vi "5_VisualAD_HyperParam_Search.vi"() -> ()   [LabVIEW 2020]
uses:
  <vilib>/Ngene/DeepLTK Anomaly Detection Addon/DeepLTK_Anomaly_Detection_Addon/API/Controls/NNPC_Coreset_Params.ctl
  <vilib>/Ngene/DeepLTK Anomaly Detection Addon/DeepLTK_Anomaly_Detection_Addon/API/Controls/NNPC_Setup.ctl
  <vilib>/Ngene/Deep Learning Toolkit/Toolkit/NN_Data/API/NN_Dims(C,H,W).ctl
  <vilib>/Ngene/Deep Learning Toolkit/Toolkit/NN_Network/Controls/NN_Device.ctl
  <vilib>/Ngene/DeepLTK Anomaly Detection Addon/DeepLTK_Anomaly_Detection_Addon/API/Controls/Feature_Scorer_Params.ctl
  <vilib>/Ngene/DeepLTK Anomaly Detection Addon/DeepLTK_Anomaly_Detection_Addon/API/Controls/Gaussian_Blur.ctl
  <vilib>/Ngene/DeepLTK Anomaly Detection Addon/DeepLTK_Anomaly_Detection_Addon/API/Controls/Evaluation_Metrics.ctl
  <vilib>/Ngene/DeepLTK Anomaly Detection Addon/DeepLTK_Anomaly_Detection_Addon/API/Controls/Eval_Results.ctl
  <vilib>/Ngene/DeepLTK Anomaly Detection Addon/DeepLTK_Anomaly_Detection_Addon/API/Controls/MinMax.ctl
  <vilib>/Ngene/DeepLTK Anomaly Detection Addon/DeepLTK_Anomaly_Detection_Addon/API/Controls/NNPC_Random_Projection_CFG.ctl
  <vilib>/Ngene/DeepLTK Anomaly Detection Addon/DeepLTK_Anomaly_Detection_Addon/API/Controls/Dim_Reduction_Method.ctl
  <vilib>/Ngene/DeepLTK Anomaly Detection Addon/DeepLTK_Anomaly_Detection_Addon/API/Controls/NNFE_CFG.ctl
  <vilib>/Ngene/DeepLTK Anomaly Detection Addon/DeepLTK_Anomaly_Detection_Addon/API/Controls/Layer_Selector.ctl
  <vilib>/Ngene/DeepLTK Anomaly Detection Addon/DeepLTK_Anomaly_Detection_Addon/API/Controls/Feature_Layer_Selector.ctl
  <vilib>/Ngene/DeepLTK Anomaly Detection Addon/DeepLTK_Anomaly_Detection_Addon/API/Controls/Interpolation_Selector.ctl
  subVIs/Dataset_Reader/Controls/Read_Options.ctl
  <vilib>/Ngene/DeepLTK Anomaly Detection Addon/DeepLTK_Anomaly_Detection_Addon/API/Controls/NNPC_PreProcessing_Options.ctl
  <vilib>/Ngene/DeepLTK Anomaly Detection Addon/DeepLTK_Anomaly_Detection_Addon/API/Controls/NNPC_DS_Stats.ctl
  <vilib>/Ngene/DeepLTK Anomaly Detection Addon/DeepLTK_Anomaly_Detection_Addon/API/Controls/Image_Stats_RGB.ctl
  subVIs/HyperParam_Investigation/Controls/Model_Info_and_Report.ctl
  subVIs/HyperParam_Investigation/Controls/Feature_Layers_CFG.ctl
  <vilib>/Ngene/DeepLTK Anomaly Detection Addon/DeepLTK_Anomaly_Detection_Addon/API/Controls/Eval_Config.ctl
  <vilib>/Ngene/Deep Learning Toolkit/Toolkit/NN_Data/subVIs/Dataset_Destroy/NN_Dataset_Destroy(In3D_Out3D).vi
  <vilib>/Ngene/DeepLTK Anomaly Detection Addon/DeepLTK_Anomaly_Detection_Addon/API/Controls/NNPC_Save_CFG.ctl
  <vilib>/Ngene/DeepLTK Anomaly Detection Addon/DeepLTK_Anomaly_Detection_Addon/API/NNPC_Generate_Embedding/NNPC_Generate_Embedding(Dataset).vi
  <vilib>/Ngene/DeepLTK Anomaly Detection Addon/DeepLTK_Anomaly_Detection_Addon/API/NNPC_Predict/NNPC_Predict(Dataset).vi
  <vilib>/Ngene/DeepLTK Anomaly Detection Addon/DeepLTK_Anomaly_Detection_Addon/DeepLTK_Anomaly_Detection_Addon.lvlib
  <vilib>/Ngene/Deep Learning Toolkit/Toolkit/Deep_Learning_Toolkit_by_Ngene.lvlib
panel:
  in  "Tab Control":enum32{"Setup", "Results"}(tab)
  in  "Max_Layers_In_1_Group":u16=2
  in  "Dataset_Path(Train/Test/GT)":path=path "D:/DNN/_AD/_from_Customers/2025_04_11_NIConnect_Cards/1_Dataset/0_Orig"
  in  "PatchCore_Dest_Folder_Path":path=path "D:/Ngene/Projects_SVN/AD/Projects/2025/2025_04_09_VAD_RT_NIConnect/Models/HPO"
  in  "Coreset_Size":sgl[](array[numeric])=[1000.0, 5000.0, 10000.0, 15000.0]
  in  "Image Res.":i32[](array[numeric])=[224, 320, 448, 480]
  in  "Proj._Dim.":i32[](array[numeric])=[-1]
  in  "Coreset_Params":T1={"CoreSet_Size"=2000.0, "Start_idx"=3}
  in  "NNPC_Setup":T2={"Input_Dims"={"C"=3, "H"=224, "W"=224}, "mBatch"=1, "Device"=enum."GPU", "GPU Id"=0}
  in  "Feature_Scorer_Params":T5={"Nearest_Neighbors"=1, "Calculate Anomaly Map"=FALSE, "Gaussian_Blur"={"Kernel_Size"=33, "Sigma"=4.0}}
  in  "Dim Reduction":T7={"Method"=enum."None", "Target_Dim"=-1, "Seed"=42}
  in  "NNFE_CFG":T9={"Name"="AD_PCB4", "Layer_Selection_By"=enum."Layer_Idx", "Feature_Layers"={"[LayerID, PatchSize]"=[{"Layer_ID"=8, "Patch_Size"=3}, {"Layer_ID"=16, "Patch_Size"=3}]}, "Interpolation_Type"=enum."Bi-Linear"}
  in  "NNFE_Folder_Paths":path[](array[path])=[path "D:/Ngene/Projects_SVN/AD/Projects/2025/2025_04_09_VAD_RT_NIConnect/VAD_Host_Train_v1.0/NNFE/RN18_2"]
  in  "Patch Sizes":i32[](array[numeric])=[1, 3, 5]
  in  "Layer IDs":i32[](array[numeric])=[15, 22]
  out "Feature_Layers":T11[](array[typedef])
  out "Max_Dist":sgl[](graph)
  out "Total Iters":i32
  out "Current Iter":i32=12
  out "Coreset Size":i32=3
  out "Proj. Dim.":i32=2
  out "Img Res.":i32=3
  out "Feature_Layers":i32=8
  out "Elapsed Time":dbl format="%<%H:%M:%S>t"
  out "Evaluation_Metrics(Image)":T13 {"Eval Stats"."Recall(F1_Max)" format="%#.5f"; "Eval Stats"."FPR(F1_Max)" format="%#.5f"; "Eval Stats"."FNR(F1_Max)" format="%#.5f"; "Eval Stats"."Prec.(F1_Max)" format="%#.5f"; "Eval Stats"."F1_Max" format="%#.5f"; "Eval Stats"."AUROC" format="%#.5f"; "Eval Stats"."Scores(Bad)"."Min" format="%#_5g"; "Eval Stats"."Scores(Good)"."Min" format="%#_5g"; "Eval Stats"."Thrshld(F1_Max)" format="%#_5f"}
  out "Evaluation_Metrics(Pixel)":T13 {"Eval Stats"."Recall(F1_Max)" format="%#.5f"; "Eval Stats"."FPR(F1_Max)" format="%#.5f"; "Eval Stats"."FNR(F1_Max)" format="%#.5f"; "Eval Stats"."Prec.(F1_Max)" format="%#.5f"; "Eval Stats"."F1_Max" format="%#.5f"; "Eval Stats"."AUROC" format="%#.5f"; "Eval Stats"."Scores(Bad)"."Min" format="%#_5g"; "Eval Stats"."Scores(Good)"."Min" format="%#_5g"; "Eval Stats"."Thrshld(F1_Max)" format="%#_5f"}
  out "Coreset Size":i32
  out "Coreset Size":sgl=15000.0
  out "Proj. Dim.":i32=256
  out "Img. Res.":i32=448
  out "Proj. Dim.":i32
  out "Img Res.":i32
  out "dT_Eval":dbl format="%#_4p"
  out "dT_Inference":dbl format="%#_4p"
  out "dT_Coreset":dbl format="%#_4p"
  out "dT_Embed":dbl format="%#_3p"
  out "dT_Init":dbl=20.247487999999976 format="%#_3p"
  out "dT_DS_Read(Test)":dbl=7.12646570000004 format="%#_3p"
  out "dT_DS_Read(Train)":dbl=7.636317299999973 format="%#_3p"
  out "DS Size(Test)":i32=600
  out "DS Size(Train)":i32=500
  out "Feature_Layers":i32
  out "error out":errorcluster
  out "dT_DS_Read(Train)":dbl
  out "dT_DS_Read(Test)":dbl
  out "dT_Init":dbl
  out "dT_Predict":dbl
  out "dT_Coreset":dbl
  out "dT_Embed":dbl
  out "dT_Eval":dbl
  out "Feature Extractor":string="wrn_50_2_2_bnmerge"
  out "dT_Predict":dbl
  out "[LayerID, PatchSize]":cluster{"Layer_ID":i32, "Patch_Size":i32}[](array[cluster])=[{"Layer_ID"=32, "Patch_Size"=1}]
  in  "Stop":bool
  out "NNFE":i32
  out "NNFE":i32
  # "Total Iterations"
  # "Current Iteration"
  # "Current Settings"
  # "Total Times"
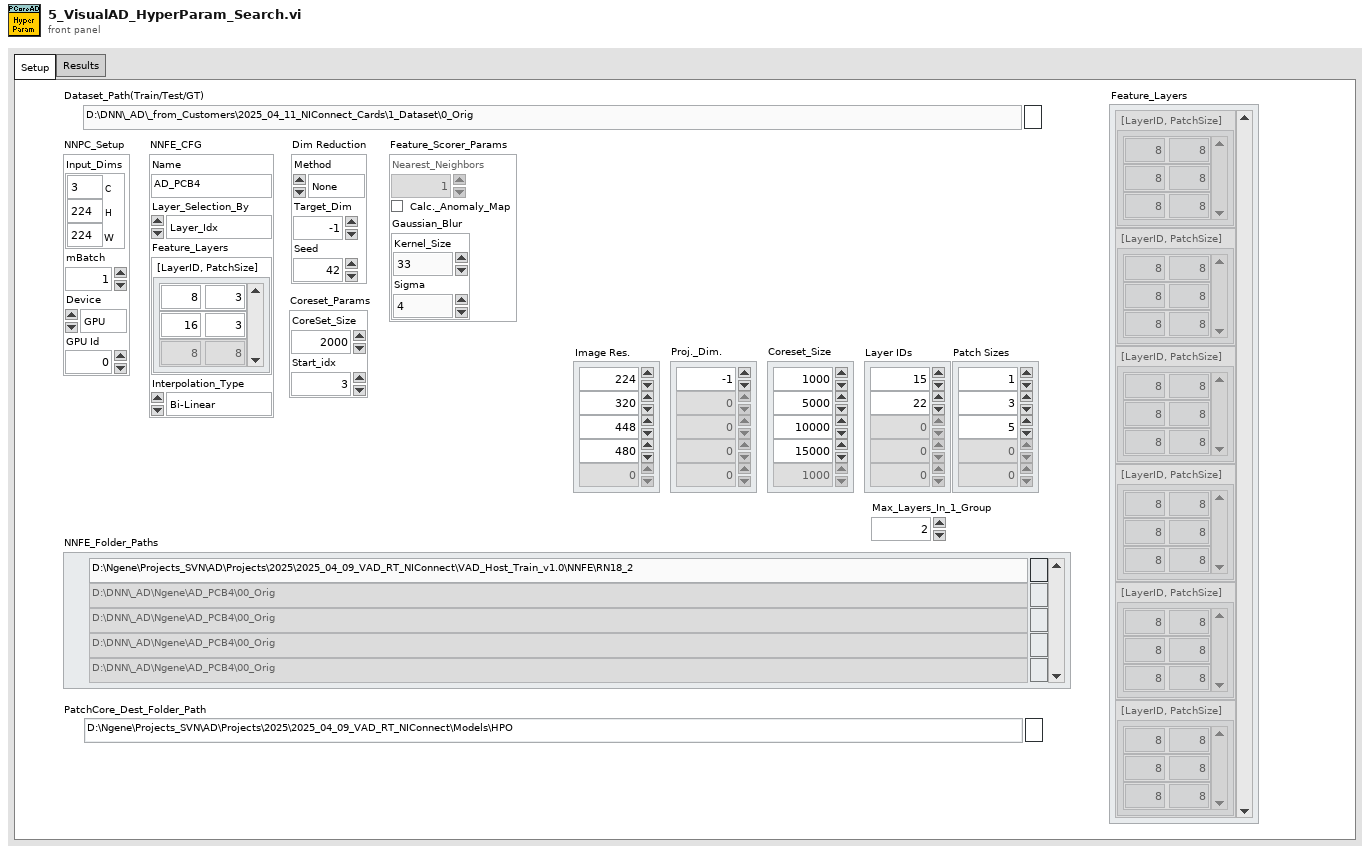
[diagram p1: front panel]
types:
  T1 = typedef "DeepLTK_Anomaly_Detection_Addon.lvlib/NNPC_Coreset_Params.ctl" = cluster{"CoreSet_Size":sgl, "Start_idx":i32}
  T2 = typedef "DeepLTK_Anomaly_Detection_Addon.lvlib/NNPC_Setup.ctl" = cluster{"Input_Dims":T3, "mBatch":i32, "Device":T4, "GPU Id":i32}
  T3 = typedef "Deep_Learning_Toolkit_by_Ngene.lvlib/NN_Dims(C,H,W).ctl" = cluster{"C":i32, "H":i32, "W":i32}
  T4 = typedef "Deep_Learning_Toolkit_by_Ngene.lvlib/NN_Device.ctl" = enum16{"CPU", "GPU"}
  T5 = typedef "DeepLTK_Anomaly_Detection_Addon.lvlib/Feature_Scorer_Params.ctl" = cluster{"Nearest_Neighbors":i32, "Calculate Anomaly Map":bool, "Gaussian_Blur":T6}
  T6 = typedef "DeepLTK_Anomaly_Detection_Addon.lvlib/Gaussian_Blur.ctl" = cluster{"Kernel_Size":i32, "Sigma":sgl}
  T7 = typedef "DeepLTK_Anomaly_Detection_Addon.lvlib/NNPC_Random_Projection_CFG.ctl" = cluster{"Method":T8, "Target_Dim":i32, "Seed":i32}
  T8 = typedef "DeepLTK_Anomaly_Detection_Addon.lvlib/Dim_Reduction_Method.ctl" = enum16{"None", "Rnd_Proj", "PCA"}
  T9 = typedef "DeepLTK_Anomaly_Detection_Addon.lvlib/NNFE_CFG.ctl" = cluster{"Name":string, "Layer_Selection_By":T10, "Feature_Layers":T11, "Interpolation_Type":T12}
  T10 = typedef "DeepLTK_Anomaly_Detection_Addon.lvlib/Layer_Selector.ctl" = enum16{"Stride", "Layer_Idx"}
  T11 = typedef "DeepLTK_Anomaly_Detection_Addon.lvlib/Feature_Layer_Selector.ctl" = cluster{"[LayerID, PatchSize]":cluster{"Layer_ID":i32, "Patch_Size":i32}[]}
  T12 = typedef "DeepLTK_Anomaly_Detection_Addon.lvlib/Interpolation_Selector.ctl" = enum16{"Nearest", "Bi-Linear"}
  T13 = typedef "DeepLTK_Anomaly_Detection_Addon.lvlib/Evaluation_Metrics.ctl" = cluster{"Scores(Good)":cluster{"X Values":dbl[], "Histogram: h(x)":i32[]}, "Scores(Bad)":cluster{"X Values":dbl[], "Histogram: h(x)":i32[]}, "Eval Stats":T14}
  T14 = typedef "DeepLTK_Anomaly_Detection_Addon.lvlib/Eval_Results.ctl" = cluster{"Scores(Good)":T15, "Scores(Bad)":T15, "# of Samples(Good)":i32, "# of Samples(Bad)":i32, "AUROC":sgl, "F1_Max":sgl, "Thrshld(F1_Max)":sgl, "Prec.(F1_Max)":sgl, "Recall(F1_Max)":sgl, "FPR(F1_Max)":sgl, "FNR(F1_Max)":sgl}
  T15 = typedef "DeepLTK_Anomaly_Detection_Addon.lvlib/MinMax.ctl" = cluster{"Min":sgl, "Max":sgl}
  T16 = typedef "DeepLTK_Anomaly_Detection_Addon.lvlib/NN_Paths.ctl" = cluster{"CFG":path, "BIN":path}
  T17 = typedef "DeepLTK_Anomaly_Detection_Addon.lvlib/NNPC_PreProcessing_Options.ctl" = cluster{"DS_Name":string, "Input_Dims":T3, "Center Crop Size":i32, "Interpolation Type":u32, "Multi-Stage_DownSample?":bool, "Dataset_Stats":T18}
  T18 = typedef "DeepLTK_Anomaly_Detection_Addon.lvlib/NNPC_DS_Stats.ctl" = cluster{"means":T19, "stds":T19}
  T19 = typedef "DeepLTK_Anomaly_Detection_Addon.lvlib/Image_Stats_RGB.ctl" = cluster{"R":sgl, "G":sgl, "B":sgl}
  T20 = typedef "Read_Options.ctl" = cluster{"Read Bads?":bool, "Read GTs?":bool, "Update. DS Stats?":bool}
  T21 = typedef "DeepLTK_Anomaly_Detection_Addon.lvlib/Eval_Config.ctl" = cluster{"Extract_Good_Pixels_from_Bad":bool, "# bins":i32}
  T22 = typedef "Model_Info_and_Report.ctl" = cluster{"Name":string, "Feature Extractor":string, "Input3D_Custom_Dims":T3, "Coreset Size":i32, "J-L Proj. Dim.":i32, "Train_Time":dbl, "Inf_Time":dbl, "Feature_Layers":T23, "Eval Stats(Image)":T14, "Eval Stats(Pixel)":T14}
  T23 = typedef "Feature_Layers_CFG.ctl" = cluster{"Layer_ID":i32, "Patch_Size":i32}[]
  T24 = typedef "DeepLTK_Anomaly_Detection_Addon.lvlib/NNPC_Save_CFG.ctl" = cluster{"Add_TimeStamp_SubFolder":bool, "Append_TimeStamp_to_FileNames":bool}
  T25 = typedef "Deep_Learning_Toolkit_by_Ngene.lvlib/NN_DataSet(In3D_Out3D).ctl" = cluster{"Dataset_Size":i32, "Dims_In":T3, "Labels":string[], "File Paths":path[], "Outputs Ref.":T26, "Inputs Ref.":variant, "Dims_Out":T3}
  T26 = typedef "Deep_Learning_Toolkit_by_Ngene.lvlib/NN_Data_ref(4D_SGL).ctl" = refnum<data-value>
  T27 = typedef "DeepLTK_Anomaly_Detection_Addon.lvlib/NNPC_Instance.ctl" = cluster{"NN":T28, "MemBank_Data":T43, "Name":string}
  T28 = typedef "Deep_Learning_Toolkit_by_Ngene.lvlib/NN.ctl" = cluster{"Name":string, "No of Layers":i32, "mBatch":i32, "Layers":T29[], "Dimty":T30, "Dims_In":T3, "Dims_Out":T3, "Working_Dir":path, "Train?":bool, "Train_Params":T31, "LR_Update_Policy":T34, "Session Data":T36, "Ground_truth":T37, "NNg_hdls":T38, "NN_Device":T4, "GPU Id":i32, "Labels":string[], "Receptive Field":T39[], "Loss_Type":T40, "Loss_Cfg_Prms":variant, "NNG_WS":T41}
  T29 = typedef "Deep_Learning_Toolkit_by_Ngene.lvlib/NN_Layer_ref.ctl" = refnum<data-value>
  T30 = typedef "Deep_Learning_Toolkit_by_Ngene.lvlib/NN_In_Out_Dim-ty.ctl" = enum8{"In1D_Out1D", "In3D_Out1D", "In3D_Out3D", "In3D_OutBBox"}
  T31 = typedef "Deep_Learning_Toolkit_by_Ngene.lvlib/NN_Train_Params.ctl" = cluster{"Optimizer":T32, "Beta_1":sgl, "Beta_2":sgl, "Weight Decay(L1)":sgl, "Weight Decay(L2)":sgl, "Data_Sampling":T33}
  T32 = typedef "Deep_Learning_Toolkit_by_Ngene.lvlib/NN_Train_Optimizer.ctl" = enum16{"SGD", "Adam", "Adagrad", "Adadelta", "RMSProp", "Nesterov"}
  T33 = typedef "Deep_Learning_Toolkit_by_Ngene.lvlib/NN_Train_Data_Sampling.ctl" = enum16{"Random", "Sequential"}
  T34 = typedef "Deep_Learning_Toolkit_by_Ngene.lvlib/NN_LR_Policy_Cfg.ctl" = cluster{"Policy_Type":T35, "LR0":dbl, "k":sgl, "WarmUp_Policy":enum16{"Step", "Ramp"}, "WarmUp_Iter":i32, "WarmUp_Ratio":sgl}
  T35 = typedef "Deep_Learning_Toolkit_by_Ngene.lvlib/NN_LR_Policy_Type.ctl" = enum16{"Manual", "Step", "Exp", "1/t"}
  T36 = typedef "Deep_Learning_Toolkit_by_Ngene.lvlib/NN_Train_Session_Data.ctl" = cluster{"Epochs":sgl, "Tot_Iter":i32, "LR":sgl, "LR_iter":i32}
  T37 = typedef "Deep_Learning_Toolkit_by_Ngene.lvlib/NN_Ground_truth.ctl" = cluster{"Y":variant}
  T38 = typedef "Deep_Learning_Toolkit_by_Ngene.lvlib/nng_cuda_handles.ctl" = cluster{"cudnn":u64, "cublas":u64, "stream":u64, "curand":u64}
  T39 = typedef "Deep_Learning_Toolkit_by_Ngene.lvlib/NN_Dims(V,H).ctl" = cluster{"V":i32, "H":i32}
  T40 = typedef "Deep_Learning_Toolkit_by_Ngene.lvlib/NN_Loss_Type.ctl" = enum16{"None", "MSE", "CrossEntropy", "YOLO_v2", "YOLO_v4"}
  T41 = typedef "Deep_Learning_Toolkit_by_Ngene.lvlib/NNG_WS.ctl" = cluster{"NNG_WS_Mem":T42, "Max_WS_Size":i64}
  T42 = typedef "Deep_Learning_Toolkit_by_Ngene.lvlib/NNg_WS_Mem_DVR.ctl" = refnum<data-value>
  T43 = typedef "DeepLTK_Anomaly_Detection_Addon.lvlib/MemBank_and_Norm_Variants.ctl" = cluster{"MemBank":variant, "MemBank Norm":variant}
  T44 = typedef "DeepLTK_Anomaly_Detection_Addon.lvlib/Evaluation_Metrics(Pixel_Image).ctl" = cluster{"Evaluation_Metrics(Pixel)":T13, "Evaluation_Metrics(Image)":T13}
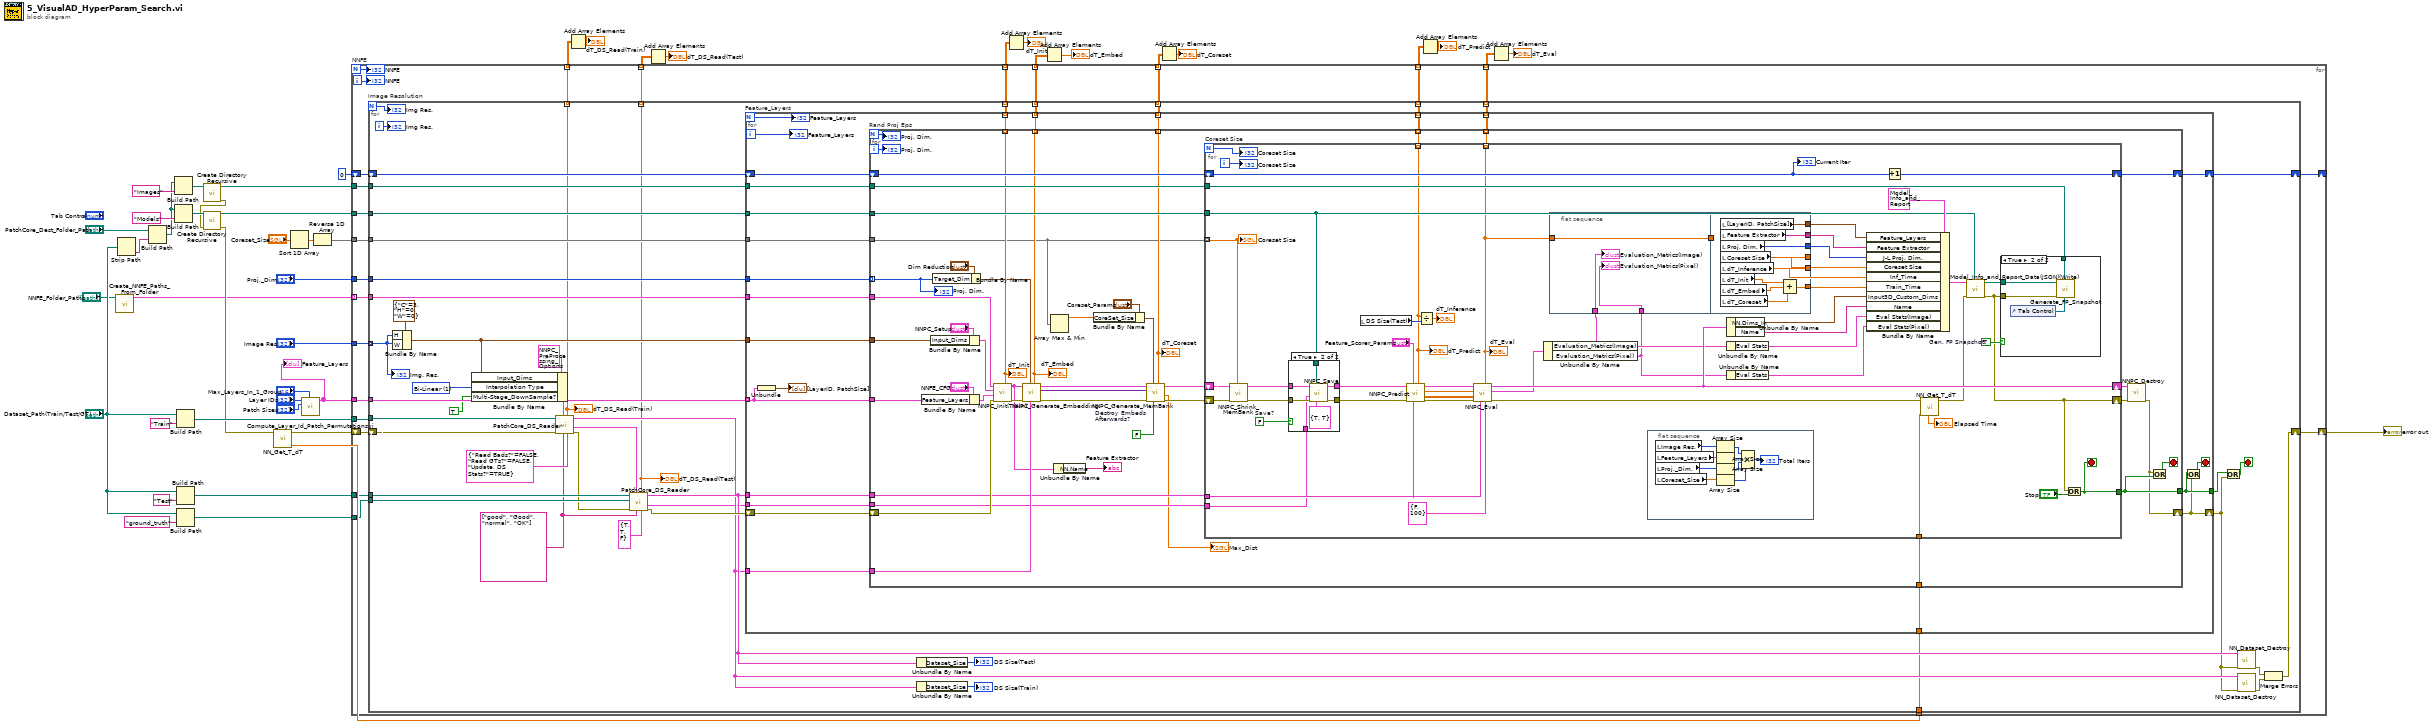
[diagram p0: block diagram]
diagram:
  n1 = call "Create_NNFE_Paths_From_Folder.vi"("NNFE_Folder_Paths"="NNFE_Folder_Paths") -> ("NNFE_File_Paths"=w9:T16[])  [unwired: 10 in]
  n2 = Strip Path(path="Dataset_Path(Train/Test/GT)") -> (name=w42:string)  [unwired: 1 out]
  n3 = Build Path(base path="PatchCore_Dest_Folder_Path", name or relative path=w42) -> (appended path=w32:path)
  n4 = Build Path(base path=w32, name or relative path="Images" ("String")) -> (appended path=w36:path)
  n5 = Build Path(base path=w32, name or relative path="Models" ("String")) -> (appended path=w35:path)
  n6 = Build Path(base path="Dataset_Path(Train/Test/GT)", name or relative path="Train" ("String")) -> (appended path=w37:path)
  n7 = Build Path(base path="Dataset_Path(Train/Test/GT)", name or relative path="Test" ("String")) -> (appended path=w38:path)
  n8 = Build Path(base path="Dataset_Path(Train/Test/GT)", name or relative path="ground_truth" ("String")) -> (appended path=w43:path)
  n9 = call <vilib>:"Create Directory Recursive.vi"("directory"=w36) -> ("error out"=w28:errorcluster, "directory copy"=w30:path)  [unwired: 4 in, 1 out]
  n10 = call <vilib>:"Create Directory Recursive.vi"("error in (no error)"=w28, "directory"=w35) -> ("error out"=w27:errorcluster, "directory copy"=w31:path)  [unwired: 3 in, 1 out]
  n11 = call <vilib>:"NN_Get_T_dT.vi"("error in (no error)"=w27) -> ("T_out"=w29:dbl, "error out"=w10:errorcluster)  [unwired: 6 in, 1 out]
  n12 = Sort 1D Array(array="Coreset_Size") -> (sorted array=w14:sgl[])
  n13 = call "Compute_Layer_Id_Patch_Permutationsvi.vi"("Limit"="Max_Layers_In_1_Group", "Patch Sizes"="Patch Sizes", "Layer IDs"="Layer IDs") -> ("LayerID,PatchSize Permutations"=w2:T11[])  [unwired: 8 in]
  "Feature_Layers" <- w2
  n14 = Reverse 1D Array(array=w14) -> (reversed array=w13:sgl[])
  n15 = for "NNFE" {
    N -> [w49]
    tunnel: "Image Res." -> [w71]
    tunnel: w43 -> [w70]
    tunnel: "Proj._Dim." -> [w69]
    tunnel: w38 -> [w68]
    tunnel: w37 -> [w67]
    tunnel: w31 -> [w66]
    tunnel: w30 -> [w65]
    tunnel: w29 -> [w64]
    tunnel: w2 -> [w63]
    tunnel: [w61] -> w25 mode=indexing
    tunnel: [w60] -> w24 mode=indexing
    tunnel: [w59] -> w23 mode=indexing
    tunnel: [w58] -> w22 mode=indexing
    tunnel: [w57] -> w21 mode=indexing
    tunnel: w13 -> [w56]
    shift-right: [w55] -> w11
    shift-left: w10 -> [w54]
    tunnel: w9 -> [w53] mode=indexing
    shift-right: [w52] -> _
    shift-left: 0 ("Img. Res. 2") -> [w62]
    tunnel: [w51] -> w7 mode=indexing
    tunnel: [w50] -> w5 mode=indexing
    i -> [w48]
    n16 = for "Image Resolution" {
      N -> [w89]
      tunnel: w70 -> [w111]
      tunnel: w67 -> [w112]
      tunnel: w71 -> [w114] mode=indexing
      tunnel: w69 -> [w116]
      tunnel: w56 -> [w115]
      tunnel: w68 -> [w110]
      shift-right: [w98] -> w55
      shift-left: w54 -> [w113]
      tunnel: w66 -> [w101]
      tunnel: w65 -> [w100]
      tunnel: w64 -> [w99]
      tunnel: w63 -> [w90]
      shift-right: [w86] -> w52
      shift-left: w62 -> [w87]
      tunnel: [w74] -> w61 mode=indexing
      tunnel: [w73] -> w60 mode=indexing
      tunnel: [w85] -> w59 mode=indexing
      tunnel: [w84] -> w51 mode=indexing
      tunnel: [w83] -> w58 mode=indexing
      tunnel: [w82] -> w57 mode=indexing
      tunnel: [w81] -> w50 mode=indexing
      tunnel: w53 -> [w75]
      i -> [w117]
      stop <- w80 stop-if-true
      w96 = u32 1 items=["Zero Order", "Bi-Linear", "Quadratic", "Cubic Spline"] ("Interpolation Type")
      w76 = string[] ["good", "Good", "normal", "OK"] ("Good Folder Name")
      n17 = Bundle By Name(cluster=T3 {"C"=3, "H"=0, "W"=0} ("Input_Dims"), "H"=w114, "W"=w114) -> (w91:T3)
      n18 = Bundle By Name(cluster=T17 {"DS_Name"="", "Input_Dims"={"C"=4, "H"=224, "W"=224}, "Center Crop Size"=-1, "Interpolation Type"=1, "Multi-Stage_DownSample?"=FALSE, "Dataset_Stats"={"means"={"R"=0.5385, "G"=0.5348, "B"=0.551}, "stds"={"R"=0.3673, "G"=0.3673, "B"=0.3505}}} ("PreProcessing_Options"), "Input_Dims"=w91, "Interpolation Type"=w96, "Multi-Stage_DownSample?"=TRUE) -> (w78:T17)
      n19 = call "PatchCore_DS_Reader.vi"("Read Options"=T20 {"Read Bads?"=FALSE, "Read GTs?"=FALSE, "Update. DS Stats?"=TRUE}, "Good Unique Labels"=w76, "PreProc_Options_in"=w78, "error in (no error)"=w113, "Folder Path"=w112) -> ("error out"=w109:errorcluster, "PreProc_Options_out"=w77:T17, "Dataset"=w103:T25, "dT_DS_Reader"=w74:dbl)  [unwired: 3 in]
      "dT_DS_Read(Train)" <- w74
      n20 = call "PatchCore_DS_Reader.vi"("Read Options"=T20 {"Read Bads?"=TRUE, "Read GTs?"=TRUE, "Update. DS Stats?"=FALSE}, "Good Unique Labels"=w76, "PreProc_Options_in"=w77, "error in (no error)"=w109, "GT Folder Path"=w111, "Folder Path"=w110) -> ("error out"=w107:errorcluster, "PreProc_Options_out"=w93:T17, "Dataset"=w104:T25, "dT_DS_Reader"=w73:dbl)  [unwired: 2 in]
      "dT_DS_Read(Test)" <- w73
      n21 = for "Feature_Layers" {
        N -> [w130]
        tunnel: w116 -> [w142]
        tunnel: w115 -> [w141]
        tunnel: w104 -> [w139]
        tunnel: w103 -> [w138]
        tunnel: w101 -> [w137]
        tunnel: w100 -> [w136]
        tunnel: w99 -> [w135]
        tunnel: w93 -> [w134]
        shift-right: [w120] -> w79
        shift-left: w107 -> [w140]
        tunnel: w91 -> [w132]
        tunnel: w90 -> [w131] mode=indexing
        tunnel: [w129] -> w88
        shift-right: [w128] -> w86
        shift-left: w87 -> [w127]
        tunnel: [w126] -> w85 mode=indexing
        tunnel: [w125] -> w84 mode=indexing
        tunnel: [w124] -> w83 mode=indexing
        tunnel: [w123] -> w82 mode=indexing
        tunnel: [w122] -> w81 mode=indexing
        tunnel: w75 -> [w118]
        i -> [w133]
        stop <- w121 stop-if-true
        n22 = Unbundle(w131) -> ("[LayerID, PatchSize]"=→"[LayerID, PatchSize]":cluster{"Layer_ID":i32, "Patch_Size":i32}[])
        n23 = for "Rand Proj Eps" {
          N -> [w170]
          tunnel: w137 -> [w187]
          tunnel: w138 -> [w182]
          tunnel: w142 -> [w177] mode=indexing
          tunnel: w141 -> [w145]
          shift-right: [w161] -> w120
          shift-left: w140 -> [w186]
          tunnel: w139 -> [w180]
          tunnel: w136 -> [w179]
          tunnel: w135 -> [w178]
          tunnel: w134 -> [w176]
          tunnel: w132 -> [w172]
          tunnel: w131 -> [w171]
          tunnel: [w169] -> w129
          shift-right: [w167] -> w128
          shift-left: w127 -> [w168]
          tunnel: [w166] -> w126 mode=indexing
          tunnel: [w165] -> w125 mode=indexing
          tunnel: [w149] -> w124 mode=indexing
          tunnel: [w164] -> w123 mode=indexing
          tunnel: [w163] -> w122 mode=indexing
          tunnel: w118 -> [w144]
          i -> [w185]
          stop <- w162 stop-if-true
          w153 = FALSE  # Destroy Embeds Afterwards?
          n24 = Bundle By Name(cluster="NNFE_CFG", "Feature_Layers"=w171) -> (w160:T9)
          n25 = Bundle By Name(cluster="NNPC_Setup", "Input_Dims"=w172) -> (w159:T2)
          n26 = Bundle By Name(cluster="Dim Reduction", "Target_Dim"=w177) -> (w158:T7)
          n27 = call <vilib>:"NNPC_Init(Train).vi"("error in"=w186, "NNFE_CFG"=w160, "NNPC_Setup"=w159, "NNFE_Paths"=w144) -> ("error out"=w183:errorcluster, "NNPC_out"=w157:T27, "dT_Init_Train"=w166:dbl)  [unwired: 5 in]
          "dT_Init" <- w166
          n28 = call-poly <vilib>:"NNPC_Generate_Embedding.vi"("Dataset"=w182, "Dim_Reduction"=w158, "error in"=w183, "NNPC_in"=w157) -> ("error out"=w152:errorcluster, "Feature_Embeddings"=w151:variant, "NNPC_out"=w150:T27, "dT_Embed"=w165:dbl)  [unwired: 3 in, 1 out]
          "dT_Embed" <- w165
          n29 = Array Max & Min(array=w145) -> (max value=w148:sgl)  [unwired: 3 out]
          n30 = Unbundle By Name(w157) -> ("NN.Name"=→"Feature Extractor":string)
          n31 = Bundle By Name(cluster="Coreset_Params", "CoreSet_Size"=w148) -> (w155:T1)
          n32 = call <vilib>:"NNPC_Generate_MemBank.vi"("Destroy Embeds Afterwards?"=w153, "Coreset_Params"=w155, "error in (no error)"=w152, "Feature_Embeddings"=w151, "NNPC_in"=w150) -> ("error out"=w147:errorcluster, "Max_Distances"=→"Max_Dist":sgl[], "NNPC_out"=w146:T27, "dT_Coreset"=w149:dbl)  [unwired: 3 in]
          "dT_Coreset" <- w149
          n33 = for "Coreset Size" {
            N -> [w209]
            tunnel: w187 -> [w217]
            shift-right: [w216] -> w184
            shift-left: w146 -> [w194]
            shift-right: [w198] -> w181
            shift-left: w147 -> [w192]
            tunnel: w180 -> [w230]
            tunnel: w179 -> [w219]
            tunnel: w178 -> [w215]
            tunnel: w176 -> [w210]
            tunnel: [w206] -> w169
            shift-right: [w202] -> w167
            shift-left: w168 -> [w203]
            tunnel: [w201] -> w164 mode=indexing
            tunnel: [w200] -> w163 mode=indexing
            tunnel: w145 -> [w190] mode=indexing
            i -> [w239]
            stop <- w206 stop-if-true
            w220 = TRUE  # Gen. FP Snapshot?
            w228 = FALSE  # Save?
            n34 = call <vilib>:"NNPC_Shrink_MemBank.vi"("Coreset_Size"=w190, "error in (no error)"=w192, "NNPC_in"=w194) -> ("error out"=w191:errorcluster, "NNPC_out"=w193:T27)  [unwired: 7 in]
            n35 = case shown="True" w228 {
              tunnel: w217 -> [_ w273]
              tunnel: w191 -> [w265 w272]
              tunnel: w193 -> [w266 w271]
              tunnel: [w265 w269] -> w231
              tunnel: [w266 w268] -> w229
              tunnel: w210 -> [_ w267]
              frame False {
              }
              frame True {
                n36 = call <vilib>:"NNPC_Save.vi"("Save_Config"=T24 {"Add_TimeStamp_SubFolder"=TRUE, "Append_TimeStamp_to_FileNames"=TRUE} ("Save Config"), "Dst_Folder"=w273, "error in (no error)"=w272, "PreProc_Options_in"=w267, "NNPC_in"=w271) -> ("error out"=w269:errorcluster, "NNPC_out"=w268:T27)  [unwired: 4 in, 1 out]
              }
            }
            n37 = local read "DS Size(Test)"() -> (w226:i32)
            n38 = call-poly <vilib>:"NNPC_Predict.vi"("Dataset"=w230, "Feature_Scorer_Params"="Feature_Scorer_Params", "error in (no error)"=w231, "NNPC_in"=w229) -> ("error out"=w234:errorcluster, "Anomaly_Maps"=w233:sgl[][][], "Pred_Scores"=w235:sgl[], "NNPC_out"=w236:T27, "dT_Predict"=w201:dbl)  [unwired: 3 in]
            "dT_Predict" <- w201
            n39 = Divide(x=w201, y=w226) -> (x/y=→"dT_Inference":dbl)
            n40 = call <vilib>:"NNPC_Eval.vi"("Eval_Config"=T21 {"Extract_Good_Pixels_from_Bad"=FALSE, "# bins"=100} ("Eval Config"), "Dataset"=w230, "error in (no error)"=w234, "Anomaly_Maps"=w233, "Pred_Scores"=w235, "NNPC_in"=w236) -> ("error out"=w208:errorcluster, "Evaluation_Metrics"=w204:T44, "NNPC_out"=w216:T27, "dT_Eval"=w200:dbl)  [unwired: 2 in]
            "dT_Eval" <- w200
            n41 = Unbundle By Name(w204) -> ("Evaluation_Metrics(Image)"=w197:T13, "Evaluation_Metrics(Pixel)"=w196:T13)
            n42 = flat-sequence {
              tunnel: w200 -> [w251]
              tunnel: [w251] -> w205
              tunnel: w196 -> [w250]
              tunnel: w197 -> [w249]
              tunnel: [w257] -> w225
              tunnel: [w256] -> w213
              tunnel: [w255] -> w212
              tunnel: [w254] -> w211
              tunnel: w205 -> [_]
              tunnel: [w253] -> w195
              tunnel: [w252] -> w189
              frame #0 {
                "Evaluation_Metrics(Image)" <- w249
                "Evaluation_Metrics(Pixel)" <- w250
              }
              frame #1 {
                n43 = local read "[LayerID, PatchSize]"() -> (w252:cluster{"Layer_ID":i32, "Patch_Size":i32}[])
                n44 = local read "Feature Extractor"() -> (w253:string)
                n45 = local read "Proj. Dim."() -> (w254:i32)
                n46 = local read "Coreset Size"() -> (w255:sgl)
                n47 = local read "dT_Inference"() -> (w256:dbl)
                n48 = local read "dT_Init"() -> (w260:dbl)
                n49 = local read "dT_Embed"() -> (w259:dbl)
                n50 = local read "dT_Coreset"() -> (w258:dbl)
                n51 = Compound Arithmetic op=ADD(w260, w259, w258) -> (w257:dbl)
              }
            }
            n52 = flat-sequence {
              frame #0 {
                n53 = local read "Image Res."() -> (w248:i32[])
                n54 = local read "Feature_Layers"() -> (w240:T11[])
                n55 = local read "Proj._Dim."() -> (w247:i32[])
                n56 = local read "Coreset_Size"() -> (w246:sgl[])
                n57 = Array Size(array=w248) -> (size(s)=w244:i32)
                n58 = Array Size(array=w240) -> (size(s)=w245:i32)
                n59 = Array Size(array=w247) -> (size(s)=w243:i32)
                n60 = Array Size(array=w246) -> (size(s)=w242:i32)
                n61 = Compound Arithmetic op=MULTIPLY(w244, w245, w243, w242) -> (→"Total Iters":i32)
              }
            }
            n62 = Unbundle By Name(w216) -> ("NN.Dims_In"=w222:T3, "Name"=w221:string)
            n63 = Unbundle By Name(w197) -> ("Eval Stats"=w224:T14)
            n64 = Unbundle By Name(w196) -> ("Eval Stats"=w223:T14)
            n65 = Bundle By Name(cluster=T22 {"Name"="", "Feature Extractor"="wrn_50_2_2_bnmerge", "Input3D_Custom_Dims"={"C"=0, "H"=0, "W"=-1}, "Coreset Size"=0, "J-L Proj. Dim."=0, "Train_Time"=0.0, "Inf_Time"=0.0, "Feature_Layers"=[{"Layer_ID"=8, "Patch_Size"=3}, {"Layer_ID"=16, "Patch_Size"=3}], "Eval Stats(Image)"={"Scores(Good)"={"Min"=0.0, "Max"=0.0}, "Scores(Bad)"={"Min"=0.0, "Max"=0.0}, "# of Samples(Good)"=0, "# of Samples(Bad)"=0, "AUROC"=0.0, "F1_Max"=0.0, "Thrshld(F1_Max)"=0.0, "Prec.(F1_Max)"=0.0, "Recall(F1_Max)"=0.0, "FPR(F1_Max)"=0.0, "FNR(F1_Max)"=0.0}, "Eval Stats(Pixel)"={"Scores(Good)"={"Min"=0.0, "Max"=0.0}, "Scores(Bad)"={"Min"=0.0, "Max"=0.0}, "# of Samples(Good)"=0, "# of Samples(Bad)"=0, "AUROC"=0.0, "F1_Max"=0.0, "Thrshld(F1_Max)"=0.0, "Prec.(F1_Max)"=0.0, "Recall(F1_Max)"=0.0, "FPR(F1_Max)"=0.0, "FNR(F1_Max)"=0.0}} ("Model_Info_and_Report"), "Feature_Layers"=w189, "Feature Extractor"=w195, "J-L Proj. Dim."=w211, "Coreset Size"=w212, "Inf_Time"=w213, "Train_Time"=w225, "Input3D_Custom_Dims"=w222, "Name"=w221, "Eval Stats(Image)"=w224, "Eval Stats(Pixel)"=w223) -> (w238:T22)
            n66 = Increment(x=w203) -> (x+1=w202:i32)
            n67 = call <vilib>:"NN_Get_T_dT.vi"("T_in"=w215, "error in (no error)"=w208) -> ("error out"=w199:errorcluster, "dT"=→"Elapsed Time":dbl)  [unwired: 5 in, 1 out]
            n68 = call "Model_Info_and_Report_Data(JSON)(Write).vi"("Dest Folder"=w217, "error in (no error)"=w199, "Model_Info_and_Report"=w238) -> ("error out"=w198:errorcluster, "Generated File Path"=w218:path)  [unwired: 7 in]
            n69 = case shown="True" w220 {
              tunnel: w219 -> [_ w262]
              tunnel: w218 -> [_ w261]
              tunnel: w198 -> [_ w263]
              frame False {
              }
              frame True {
                n70 = control-ref of="Tab Control"() -> (w264:refnum<vi>)
                n71 = call "Generate_FP_Snapshot.vi"("TabControl in"=w264, "directory copy"=w262, "error in"=w263, "Generated File Path"=w261) -> ()  [unwired: 7 in, 1 out]
              }
            }
            n72 = Or(x=w198, y="Stop") -> (x .or. y?=w206:bool)
            "Coreset Size" <- w239
            "Coreset Size" <- w209
            "Current Iter" <- w203
            "Coreset Size" <- w190
          }
          n73 = call <vilib>:"NNPC_Destroy.vi"("error in"=w181, "NNPC_in"=w184) -> ("error out"=w161:errorcluster)  [unwired: 9 in]
          n74 = Or(x=w161, y=w169) -> (x .or. y?=w162:bool)
          "Proj. Dim." <- w185
          "Proj. Dim." <- w177
          "Proj. Dim." <- w170
        }
        n75 = Or(x=w129, y=w120) -> (x .or. y?=w121:bool)
        "Feature_Layers" <- w133
        "Feature_Layers" <- w130
      }
      n76 = Unbundle By Name(w104) -> ("Dataset_Size"=→"DS Size(Test)":i32)
      n77 = Unbundle By Name(w103) -> ("Dataset_Size"=→"DS Size(Train)":i32)
      n78 = Or(x=w88, y=w79) -> (x .or. y?=w80:bool)
      n79 = call-poly <vilib>:"NN_Dataset_Destroy.vi"("error in (no error)"=w79, "Dataset(In3D_Out3D)"=w104) -> ("error out"=w108:errorcluster)  [unwired: 9 in]
      n80 = call-poly <vilib>:"NN_Dataset_Destroy.vi"("error in (no error)"=w79, "Dataset(In3D_Out3D)"=w103) -> ("error out"=w102:errorcluster)  [unwired: 9 in]
      n81 = Merge Errors(w108, w102) -> (w98:errorcluster)
      "Img Res." <- w117
      "Img. Res." <- w114
      "Img Res." <- w89
    }
    "NNFE" <- w49
    "NNFE" <- w48
  }
  "error out" <- w11
  n82 = Add Array Elements(numeric array=w25) -> (sum=→"dT_DS_Read(Train)":dbl)
  n83 = Add Array Elements(numeric array=w24) -> (sum=→"dT_DS_Read(Test)":dbl)
  n84 = Add Array Elements(numeric array=w23) -> (sum=→"dT_Init":dbl)
  n85 = Add Array Elements(numeric array=w7) -> (sum=→"dT_Embed":dbl)
  n86 = Add Array Elements(numeric array=w22) -> (sum=→"dT_Coreset":dbl)
  n87 = Add Array Elements(numeric array=w21) -> (sum=→"dT_Predict":dbl)
  n88 = Add Array Elements(numeric array=w5) -> (sum=→"dT_Eval":dbl)
